vi "Write Delayed ARINC Words.vi"() -> ()   [LabVIEW 8.6]
uses:
  <libdir>/resource/objmgr/ueidaq.rc
  vi.lib/UeiDaq/UeiDaqCreateARINCOutputSession.vi
  vi.lib/UeiDaq/UeiDaqConfigureTimingForMessagingIO.vi
panel:
  in  "TX Delay (us)":dbl
  in  "Bits per second":i32(ring) items=["12500", "100000"]
  in  "Words":T1(array[cluster])
  in  "Send":bool
  out "return count":i32
  out "device name":string
  in  "Resource":string
  out "Total words sent":i32
  in  "Refresh rate (ms)":u32
  in  "stop":bool
  # "WRITE DELAYED WORDS TO ARINC-429 PORT"
  # "1/ Set the resource name -->"
  # "2/ Set the update rate -->"
  # "Device info"
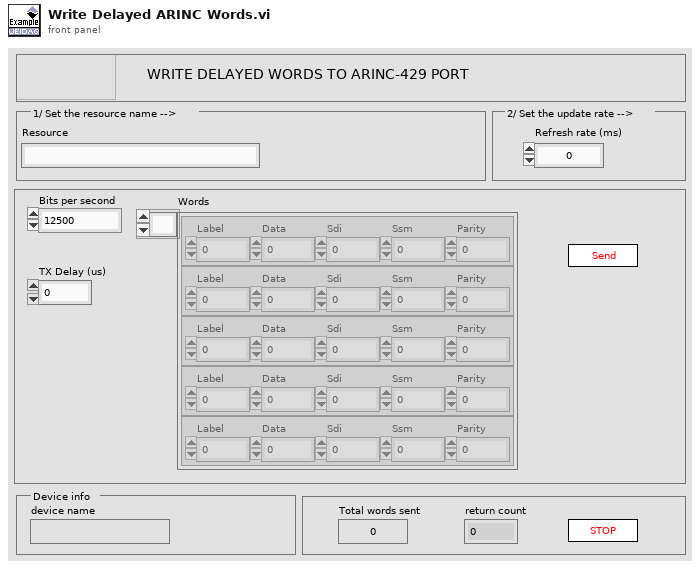
[diagram p1: front panel]
types:
  T1 = cluster{"Label":u16, "Data":u32, "Sdi":u8, "Ssm":u8, "Parity":u8}[]
  T2 = cluster{"Words":cluster{"Label":u16, "Data":u32, "Sdi":u8, "Ssm":u8, "Parity":u8}[], "TX Delay (us)":dbl}
  T3 = cluster{"Words":cluster{"Label":u16, "Data":u32, "Sdi":u8, "Ssm":u8, "Parity":u8}[], "TX Delay (us)":dbl}[]
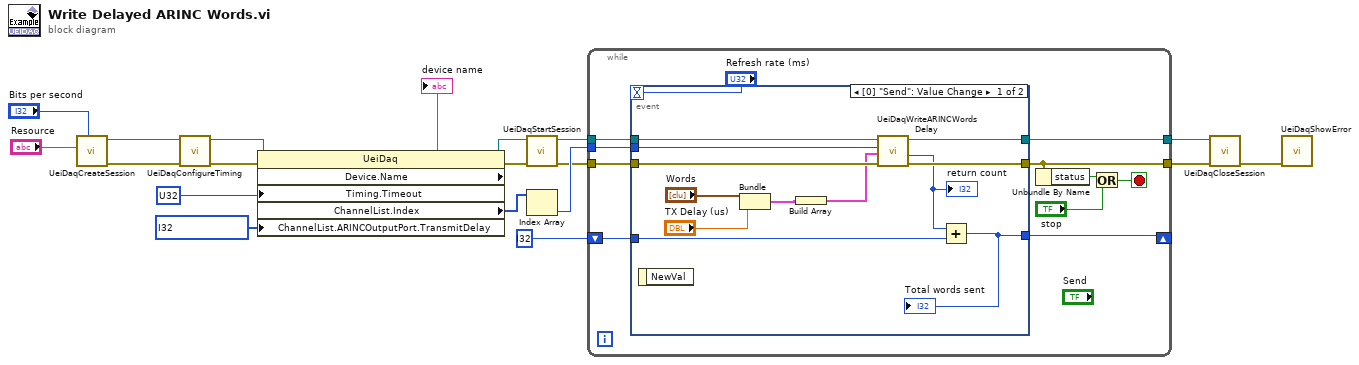
[diagram p0: block diagram]
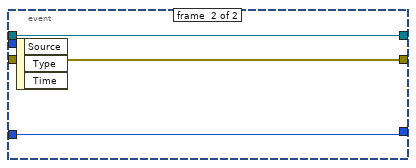
[diagram p2: hidden frame]
diagram:
  w1 = i32[] ? items=["Disable", "Enable"] ("Channel List:ARINC Output Port:TransmitDelay")
  n1 = call-poly "UeiDaqCreateSession.vi"("Bits per second"="Bits per second", "Resource"="Resource") -> ("error out"=w17:errorcluster, "UeiDaq Refnum Out"=w18:refnum<k20>)  [unwired: 4 in, 4 out]
  n2 = call-poly "UeiDaqConfigureTiming.vi"("error in (no error)"=w17, "UeiDaq Refnum In"=w18) -> ("error out"=w14:errorcluster, "UeiDaq Refnum Out"=w15:refnum<k20>)  [unwired: 2 in, 6 out]
  n3 = property class="UeiDaq"(reference=w15, error in=w14, "Timing.Timeout"=u32 ? ("Timing:Timeout"), "ChannelList.ARINCOutputPort.TransmitDelay"=w1) -> (reference out=w2:refnum<k20>, error out=w5:errorcluster, "Device.Name"=→"device name":string, "ChannelList.Index"=w7:i32[])
  n4 = call "UeiDaqStartSession.vi"("error in (no error)"=w5, "UeiDaq Refnum In"=w2) -> ("error out"=w4:errorcluster, "UeiDaq Refnum Out"=w3:refnum<k20>)  [unwired: 8 in]
  n5 = Index Array(array=w7) -> (element=w6:i32)  [unwired: 1 in]
  n6 = while {
    tunnel: w3 -> [w29]
    tunnel: w4 -> [w30]
    tunnel: [w24] -> w13
    tunnel: [w25] -> w12
    shift-right: [w22] -> _
    shift-left: i32 ? -> [w23]
    tunnel: w6 -> [w20]
    stop <- w26 stop-if-true
    n7 = event shown="[0] \"Send\": Value Change" {
      selector: _ -> [_ _]
      dyn-events: _ -> [_ _]
      timeout: "Refresh rate (ms)" -> [_ _]
      tunnel: w30 -> [w42 w44]
      tunnel: w29 -> [w41 w45]
      tunnel: [w40 w45] -> w25
      tunnel: [w39 w44] -> w24
      tunnel: w23 -> [w37 w43]
      tunnel: [w36 w43] -> w22
      tunnel: w20 -> [w35 _]
      event #0 {
        n8 = event-data() -> ()  [unwired: 2 out]
        n9 = Bundle("Words"="Words", "TX Delay (us)"="TX Delay (us)") -> (w32:T2)  [unwired: 1 in]
        n10 = Build Array(w32) -> (w31:T3)
        n11 = call "UeiDaqWriteARINCWordsDelay.vi"("error in (no error)"=w42, "Words with Delay"=w31, "Port"=w35, "UeiDaq Refnum In"=w41) -> ("error out"=w39:errorcluster, "return count"=w38:i32, "UeiDaq Refnum Out"=w40:refnum<k20>)  [unwired: 5 in]
        "return count" <- w38
        n12 = Add(x=w38, y=w37) -> (x+y=w36:i32)
        "Total words sent" <- w36
      }
      event #1 {
        n13 = event-data() -> ()  [unwired: 4 out]
      }
    }
    n14 = Unbundle By Name(w24) -> ("status"=w28:bool)
    n15 = Or(x=w28, y="stop") -> (x .or. y?=w26:bool)
  }
  n16 = call "UeiDaqCloseSession.vi"("error in (no error)"=w13, "UeiDaq Refnum In"=w12) -> ("error out"=w19:errorcluster)  [unwired: 1 in, 8 out]
  n17 = call "UeiDaqShowError.vi"("error in (no error)"=w19) -> ()  [unwired: 2 in, 9 out]
